vi "Write to OPC Server2.vi"() -> ()   [LabVIEW 2017]
panel:
  in  "Stop Button":bool
  in  "Numeric Control":dbl=22.0
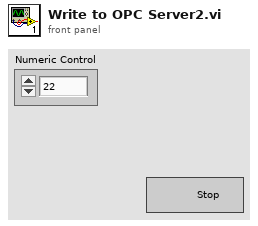
[diagram p1: front panel]
types:
  T1 = enum16{"Read", "Write", "ReadWrite", "BufferedRead", "BufferedReadWrite"}
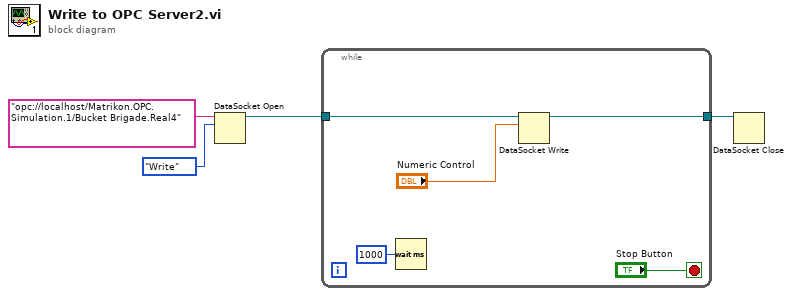
[diagram p0: block diagram]
diagram:
  n1 = DataSocket Open(10:T1."Write" ("mode"), 11:"opc://localhost/Matrikon.OPC.Simulation.1/Bucket Brigade.Real4" ("OPC URL")) -> (3:w4:refnum<k13>)  [unwired: 2 in, 1 out]
  n2 = while {
    tunnel: w4 -> [w7]
    tunnel: [w6] -> w3
    stop <- "Stop Button" stop-if-true
    n3 = Wait (ms)(milliseconds to wait=u32 1000) -> ()  [unwired: 1 out]
    n4 = DataSocket Write(10:"Numeric Control", 11:w7) -> (3:w6:refnum<k13>)  [unwired: 2 in, 2 out]
  }
  n5 = DataSocket Close(11:w3) -> ()  [unwired: 2 in, 2 out]
